vi "SeqMgr.Sequence Load Top Level Sequence, Ouput Lines.vi"(7 "Search Folders":path[](array[path]), 8 "Error In":errorcluster, 11 "Top Script File":path) -> (0 "Error Out":errorcluster, 3 "Lines Output":string[](array[string]))   [LabVIEW 2024, in "EQMF.lvlib" / "SeqMgr.lvlib"]
doc: "This VI will open the file or folder specified by the input path.\n\nIf the file or folder does not exist, this VI will indicate an error."
uses:
  SeqMgr.lvlib
panel:
  # "Reads a script\nInserts contents of file with source(Path) replaced\nwitht he text of the sourced files."
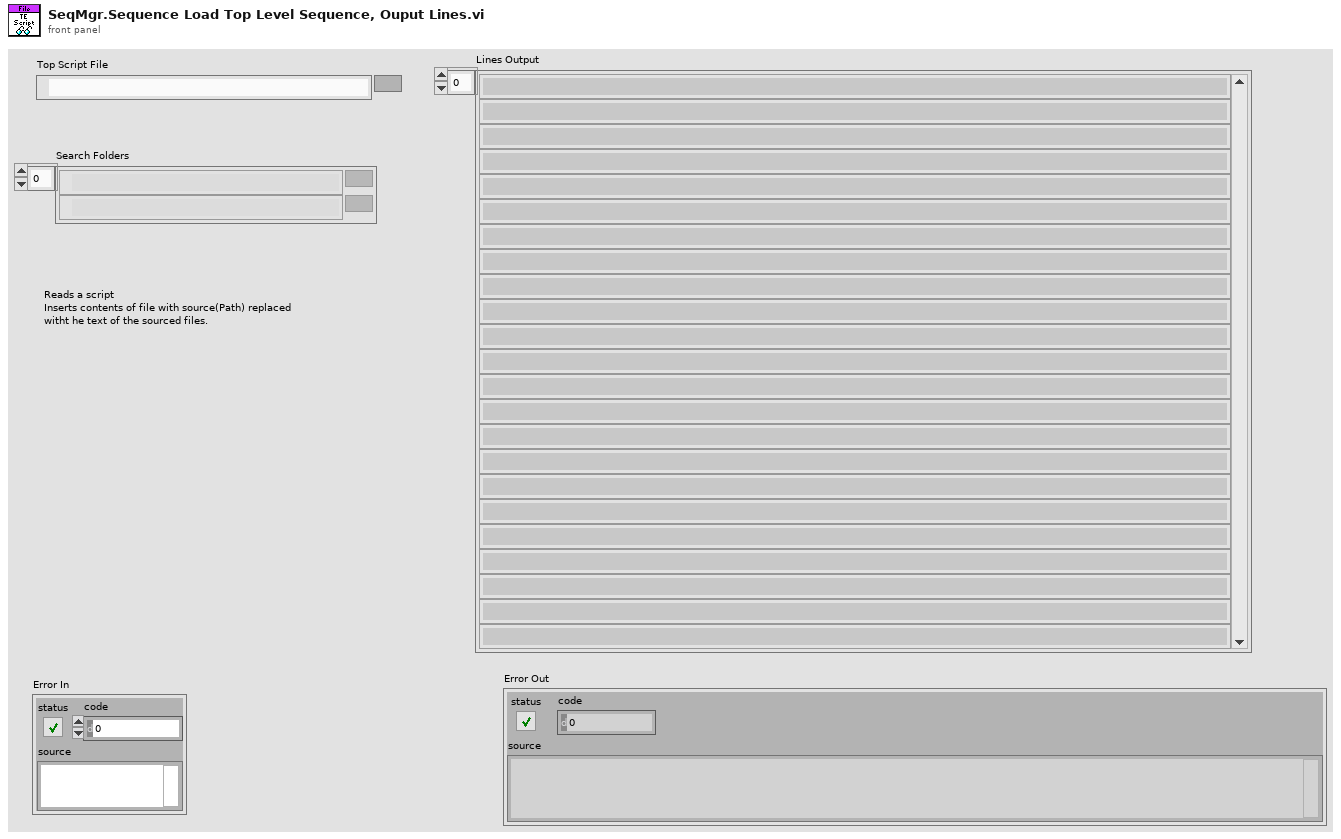
[diagram p1: front panel]
types:
  T1 = cluster{"Top Script File":path, "SearchDirs":path[], "Lines":string[]}
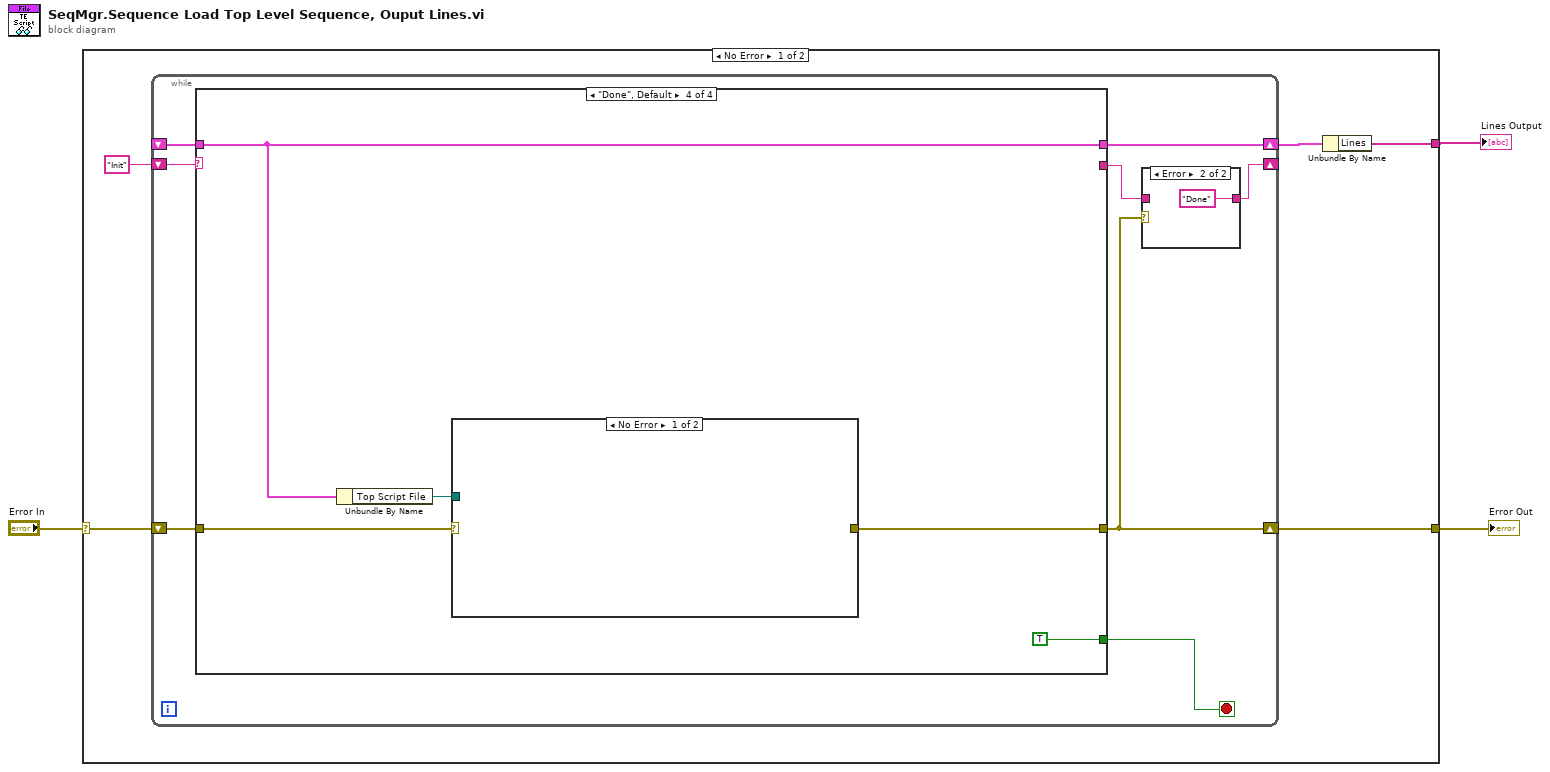
[diagram p0: block diagram]
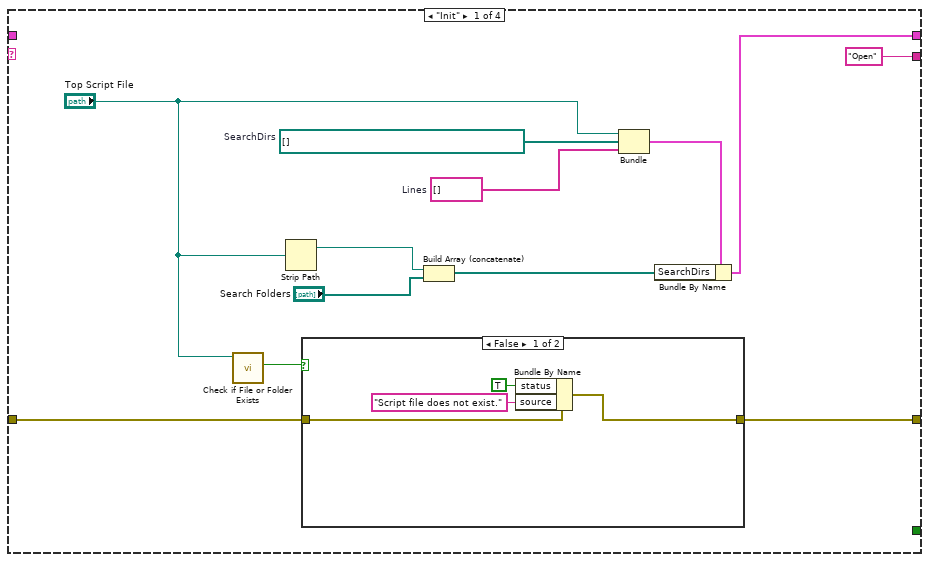
[diagram p3: hidden frame]
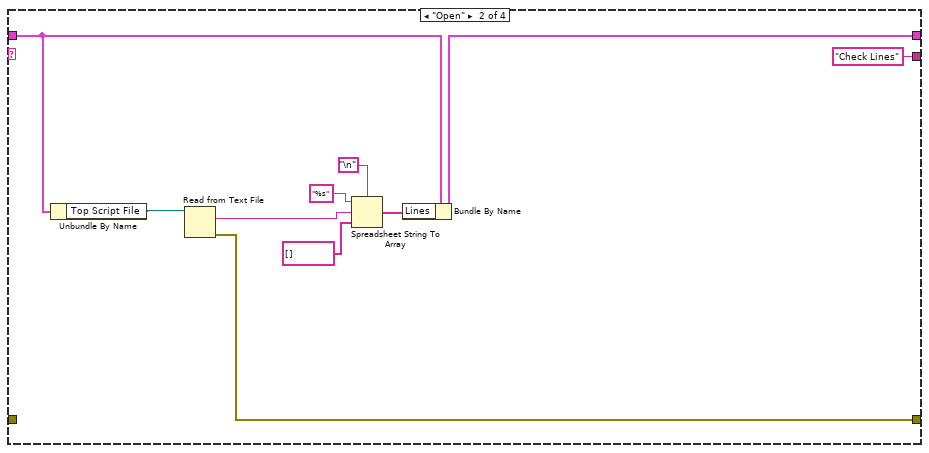
[diagram p5: hidden frame]
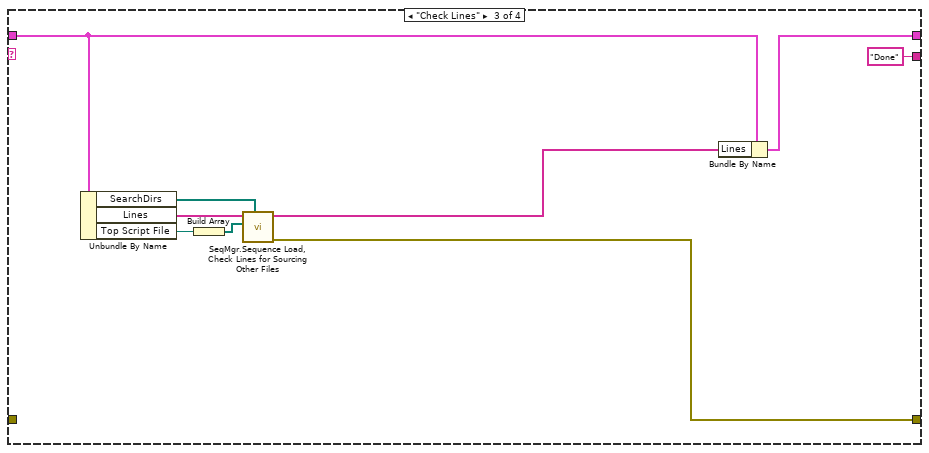
[diagram p6: hidden frame]
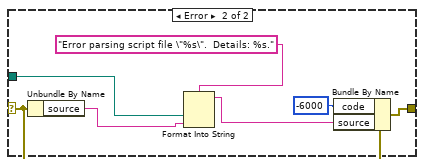
[diagram p7: hidden frame]
diagram:
  n1 = case shown="No Error" "Error In" {
    selector: "Error In" -> [w8 w67]
    tunnel: [w4 w67] -> w3
    tunnel: [w5 _] -> w1
    frame No Error {
      n2 = while {
        shift-right: [w16] -> w6
        shift-left: _ -> [w14]
        shift-right: [w10] -> _
        shift-left: "Init" -> [w15]
        shift-right: [w12] -> w4
        shift-left: w8 -> [w13]
        stop <- w9 stop-if-true
        n3 = case shown="\"Done\", Default" w15 {
          tunnel: [w24 w44 w54 w57] -> w16
          tunnel: ["Open" "Check Lines" "Done" _] -> w11
          tunnel: w14 -> [_ w43 w53 w57]
          tunnel: w13 -> [w20 _ _ w58]
          tunnel: [w19 w42 w49 w55] -> w12
          tunnel: [_ _ _ TRUE] -> w9
          frame "Init" {
            w23 = string[] []  # Lines
            w28 = path[] []  # SearchDirs
            n4 = call <vilib>:"Check if File or Folder Exists.vi"("path"="Top Script File") -> ("file or folder exists?"=w21:bool)  [unwired: 8 in, 2 out]
            n5 = Strip Path(path="Top Script File") -> (stripped path=w30:path)  [unwired: 1 out]
            n6 = case shown="False" w21 {
              tunnel: w20 -> [w34 w35]
              tunnel: [w33 w35] -> w19
              frame False {
                n7 = Bundle By Name(cluster=w34, "status"=TRUE, "source"="Script file does not exist.") -> (w33:errorcluster)
              }
              frame True {
              }
            }
            n8 = Build Array (concatenate)(w30, "Search Folders") -> (w27:path[])
            n9 = Bundle("Top Script File"="Top Script File", "SearchDirs"=w28, "Lines"=w23) -> (w25:T1)  [unwired: 1 in]
            n10 = Bundle By Name(cluster=w25, "SearchDirs"=w27) -> (w24:T1)
          }
          frame "Open" {
            n11 = Unbundle By Name(w43) -> ("Top Script File"=w45:path)
            n12 = Read from Text File(file (use dialog)=w45) -> (text=w36:string, error out=w42:errorcluster)  [unwired: 3 in, 2 out]
            n13 = Spreadsheet String To Array(delimiter (Tab)="\n", format string="%s", spreadsheet string=w36, array type (2D Dbl)=string[] []) -> (array=w37:string[])
            n14 = Bundle By Name(cluster=w43, "Lines"=w37) -> (w44:T1)
          }
          frame "Check Lines" {
            n15 = Unbundle By Name(w53) -> ("SearchDirs"=w48:path[], "Lines"=w51:string[], "Top Script File"=w47:path)
            n16 = Build Array(w47) -> (w46:path[])
            n17 = call "SeqMgr.Sequence Load, Check Lines for Sourcing Other Files.vi"("Search Folders"=w48, "Parent Scripts"=w46, "Lines In"=w51) -> ("error out"=w49:errorcluster, "Lines Out"=w50:string[])  [unwired: 7 in]
            n18 = Bundle By Name(cluster=w53, "Lines"=w50) -> (w54:T1)
          }
          frame "Done", Default {
            n19 = Unbundle By Name(w57) -> ("Top Script File"=w56:path)
            n20 = case shown="No Error" w58 {
              selector: w58 -> [_ w63]
              tunnel: w56 -> [_ w65]
              tunnel: [_ w60] -> w55
              frame No Error {
              }
              frame Error {
                n21 = Unbundle By Name(w63) -> ("source"=w64:string)
                n22 = Format Into String(format string="Error parsing script file \"%s\".  Details: %s.", w65, w64) -> (resulting string=w61:string)  [unwired: 2 in, 1 out]
                n23 = Bundle By Name(cluster=w63, "code"=-6000, "source"=w61) -> (w60:errorcluster)
              }
            }
          }
        }
        n24 = case shown="Error" w12 {
          tunnel: w11 -> [w17 _]
          tunnel: [w17 "Done"] -> w10
          frame No Error {
          }
          frame Error {
          }
        }
      }
      n25 = Unbundle By Name(w6) -> ("Lines"=w5:string[])
    }
    frame Error {
    }
  }
  "Error Out" <- w3
  "Lines Output" <- w1
